vi "DAQmx.Get Channel Map.vi"(8 "error in (no error)":errorcluster, 11 "tasks in":refnum<k21>[](array[refnum])) -> (0 "error out":errorcluster, 2 "Channel Map":T1[](array[typedef]), 3 "tasks out":refnum<k21>[](array[refnum]))   [LabVIEW 2019, in "DAQmx.lvclass"]
uses:
  DAQmx.lvclass
  typedefs/DAQmx.Channel Map--Cluster.ctl
  <resource>/objmgr/daqmx.rc
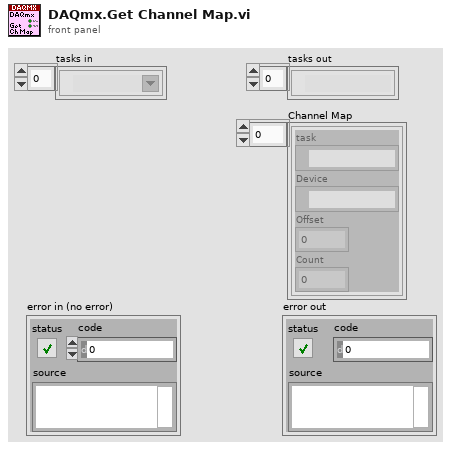
[diagram p1: front panel]
types:
  T1 = typedef "DAQmx.lvclass/DAQmx.Channel Map--Cluster.ctl" = cluster{"task":refnum<k21>, "Device":tag, "Offset":u32, "Count":u32}
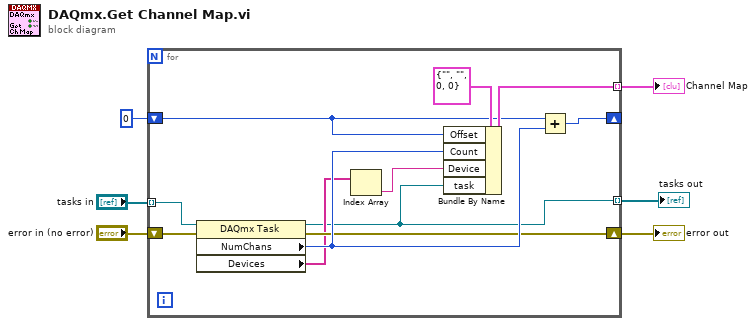
[diagram p0: block diagram]
diagram:
  n1 = for {
    shift-right: [w12] -> w2
    shift-left: "error in (no error)" -> [w17]
    tunnel: "tasks in" -> [w9] mode=indexing
    shift-right: [w14] -> _
    shift-left: u32 0 -> [w10]
    tunnel: [w13] -> w3 mode=indexing
    tunnel: [w7] -> w1 mode=indexing
    n2 = property class="DAQmx Task"(reference=w9, error in=w17) -> (reference out=w7:refnum<k21>, error out=w12:errorcluster, "NumChans"=w15:u32, "Devices"=w8:tag[])
    n3 = Index Array(array=w8) -> (element=w11:tag)  [unwired: 1 in]
    n4 = Bundle By Name(cluster=T1 {"task"="", "Device"="", "Offset"=0, "Count"=0} ("output cluster"), "Offset"=w10, "Count"=w15, "Device"=w11, "task"=w7) -> (w13:T1)
    n5 = Add(x=w10, y=w15) -> (x+y=w14:u32)
  }
  "error out" <- w2
  "Channel Map" <- w3
  "tasks out" <- w1
